vi "IMU and RoboteQ.vi"() -> ()   [LabVIEW 2012]
uses:
  LabVIEW Library v2/AHRS/Controls/Desciptor Set Byte.ctl
  <vilib>/Platform/TimedLoop/XDataNode/timing_clust.ctl
  <vilib>/Platform/TimedLoop/XDataNode/nitl_modes.ctl
  <vilib>/Platform/TimedLoop/XDataNode/wakeup.ctl
  <vilib>/FPGAPlugInAG/cRIO-9113/niLvFpga_Open_cRIO-9113.vi
  <vilib>/FPGAPlugInAG/cRIO-9113/niLvFpga_Reset_cRIO-9113.vi
  <vilib>/FPGAPlugInAG/cRIO-9113/niLvFpga_Run_cRIO-9113.vi
  <vilib>/Utility/error.llb/Error Cluster From Error Code.vi
  <vilib>/RVI Host/nirviSupport.llb/nirviErrorClusterFromErrorCode.vi
  <vilib>/rvi/errors/niLvFpgaAdjustHostInterfaceError.vi
  <vilib>/Instr/_visa.llb/VISA Configure Serial Port (Instr).vi
  LabVIEW Library v2/AHRS/SubVI/3DM-GX3-45 Commands/Start Stream.vi
  LabVIEW Library v2/AHRS/SubVI/3DM-GX3-45 Commands/Stop Stream.vi
  <vilib>/Platform/TimedLoop/XDataNode/XDataNode.xnode
  <vilib>/rvi/interface/nirviOpenFPGA/nirviOpenFPGA.xnode
  FPGA Bitfiles/NI-987xSerialLoo_FPGATarget4_9870InterfaceDMA_U4jeboZBP6A.lvbitx
  Program Files (x86)/National Instruments/LabVIEW 2012/examples/CompactRIO/Module Specific/NI 987x/Serial Loopback/VIs/9870 Interface DMA (FPGA).vi
  <vilib>/rvi/interface/nirviMethod/nirviMethod.xnode
  Labview/Roboteq.lvlib
  <vilib>/Platform/TimedLoop/XDataNode/XDNodeRunTimeDep.lvlib
  Labview/Public/Set Control Effort.vi
  <vilib>/rvi/interface/nirviMethod/StockFPGA_InlinedMethodWaitForSingleIRQ.vi
  <vilib>/FPGAPlugInAG/cRIO-9113/niLvFpga_WaitOnIrq_cRIO-9113.vi
panel:
  out "Byte Count":u32
  out "Read Bytes":string
  out "result":bool
  in  "IMU VISA":refnum<visa-resource-name>="COM5"
  out "Error Out":errorcluster
  in  "Error In":errorcluster
  out "Received Array":u8[](array[numeric]) format="%02x"
  out "Processing Loop Count":i32
  out "Received array Size":i32
  out "YAW":dbl(knob) scale=-180.0..180.0
  out "result string":string
  out "Read Loop Count":i32
  in  "Stop Data Stream":bool
  in  "Start Data Stream":bool
  in  "Self Test":bool
  out "Serial Settings:Number of Bytes at Serial Port":u32
  out "timed out?":bool
  in  "Field Data":u8[](array[numeric]) format="%02x"
  in  "Field Descriptor Byte":u8=117 format="%02x"
  in  "Data Set":T1=enum."NAV"
  in  "ID Query (True)":bool=TRUE
  in  "Motor1 Effort":i32(slide) scale=-10.0..10.0
  in  "Motor2 Effort":i32(slide) scale=-10.0..10.0
  in  "End Loop":bool
  in  "stop?":bool
  out "Telemetry":T2={"Voltage"={0.0, 0.0, 0.0}, "Encoder Speed"={0, 0}, "Temps"={"IC Temp (C)"=0, "Ch1 Temp (C)"=0, "Ch2 Temp (C)"=0}, "Current"={0.0, 0.0, 0.0, 4.6238981750249924e+36}} {"Current" scale=0.0..16.0; "Temps"."IC Temp (C)" scale=0.0..150.0; "Temps"."Ch1 Temp (C)" scale=0.0..150.0; "Temps"."Ch2 Temp (C)" scale=0.0..150.0; "Encoder Speed" scale=-100.0..100.0; "Voltage" scale=8.0..14.0}
  out "Command to Serial":string
  in  "RoboteQ VISA":refnum<visa-resource-name>
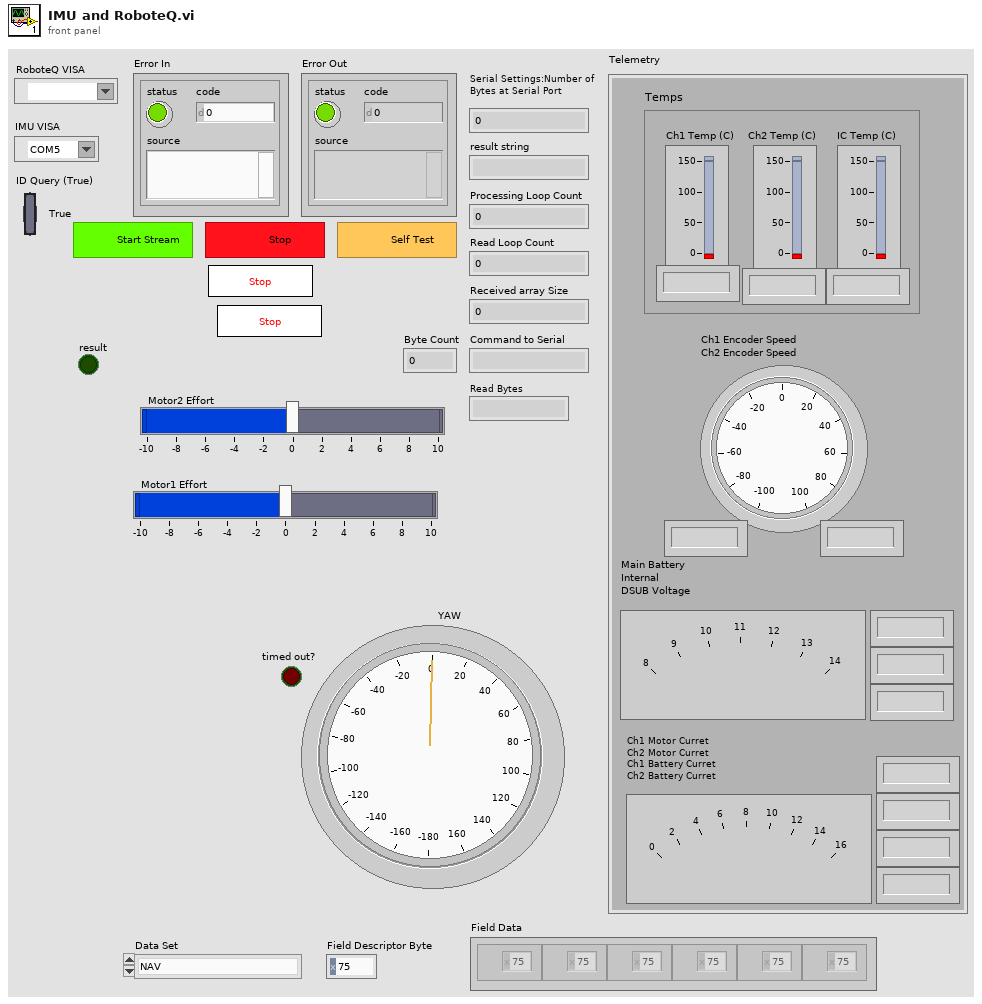
[diagram p1: front panel]
types:
  T1 = typedef "Desciptor Set Byte.ctl" = enum16{"Base Command Set", "3DM Command Set", "Navigation Filter Command Set", "System Command Set", "AHRS", "GPS", "NAV"}
  T2 = cluster{"Voltage":cluster{sgl, sgl, sgl}, "Encoder Speed":cluster{i32, i32}, "Temps":cluster{"IC Temp (C)":i32, "Ch1 Temp (C)":i32, "Ch2 Temp (C)":i32}, "Current":cluster{dbl, dbl, dbl, dbl}}
  T3 = typedef "XDNodeRunTimeDep.lvlib/timing_clust.ctl" = cluster{"Expected End [f-1]":u64, "Actual End [f-1]":u64, "Finished Late? [f-1]":bool, "Expected End [i-1]":u64, "Actual End [i-1]":u64, "Finished Late? [i-1]":bool, "Expected Start [i]":u64, "Actual Start [i]":u64, "Expected Start [f]":u64, "Actual Start [f]":u64, "Source Name":string, "Structure Name":string, "Period":i64, "Deadline":i64, "Offset":i64, "Start":i64, "Priority":i32, "Timeout":i32, "Mode":T4, "Wakeup Reason":T5, "Error":errorcluster, "Source Type":string, "Secondary Source Type":string, "Global End Time":u64, "Global Start Time":u64, "Frame Duration":u64, "Iteration Duration":u64, "Assigned CPU":i32, "I/O Scan Engine Mode":u32}
  T4 = typedef "XDNodeRunTimeDep.lvlib/nitl_modes.ctl" = enum32{"No Change", "Process missed periods, maintain original phase", "Discard missed periods, maintain original phase", "Process missed periods, ignore original phase", "Discard missed periods, ignore original phase"}
  T5 = typedef "XDNodeRunTimeDep.lvlib/wakeup.ctl" = enum32{"Normal", "Aborted", "Asynchronous wakeup", "Timing source error", "Timed loop error", "Timeout"}
  T6 = typedef "901x DMA FPGA Reference.ctl" = refnum<k20>
  T7 = cluster{"main battery voltage (V)":sgl, "internal voltage (V)":sgl, "DSUB voltage (V)":sgl}
  T8 = cluster{" Ch1  Motor current (I)":sgl, " Ch2 Motor current (I)":sgl, " Ch1 Battery current (I)":sgl, " Ch2 Battery current (I)":sgl}
  T9 = cluster{"Ch1 Temp (C)":i32, "Ch2 Temp (C)":i32, "IC Temp (C)":i32}
  T10 = cluster{"Encoder Speed (RPM)":i32, "Encoder Speed (RPM)":i32}
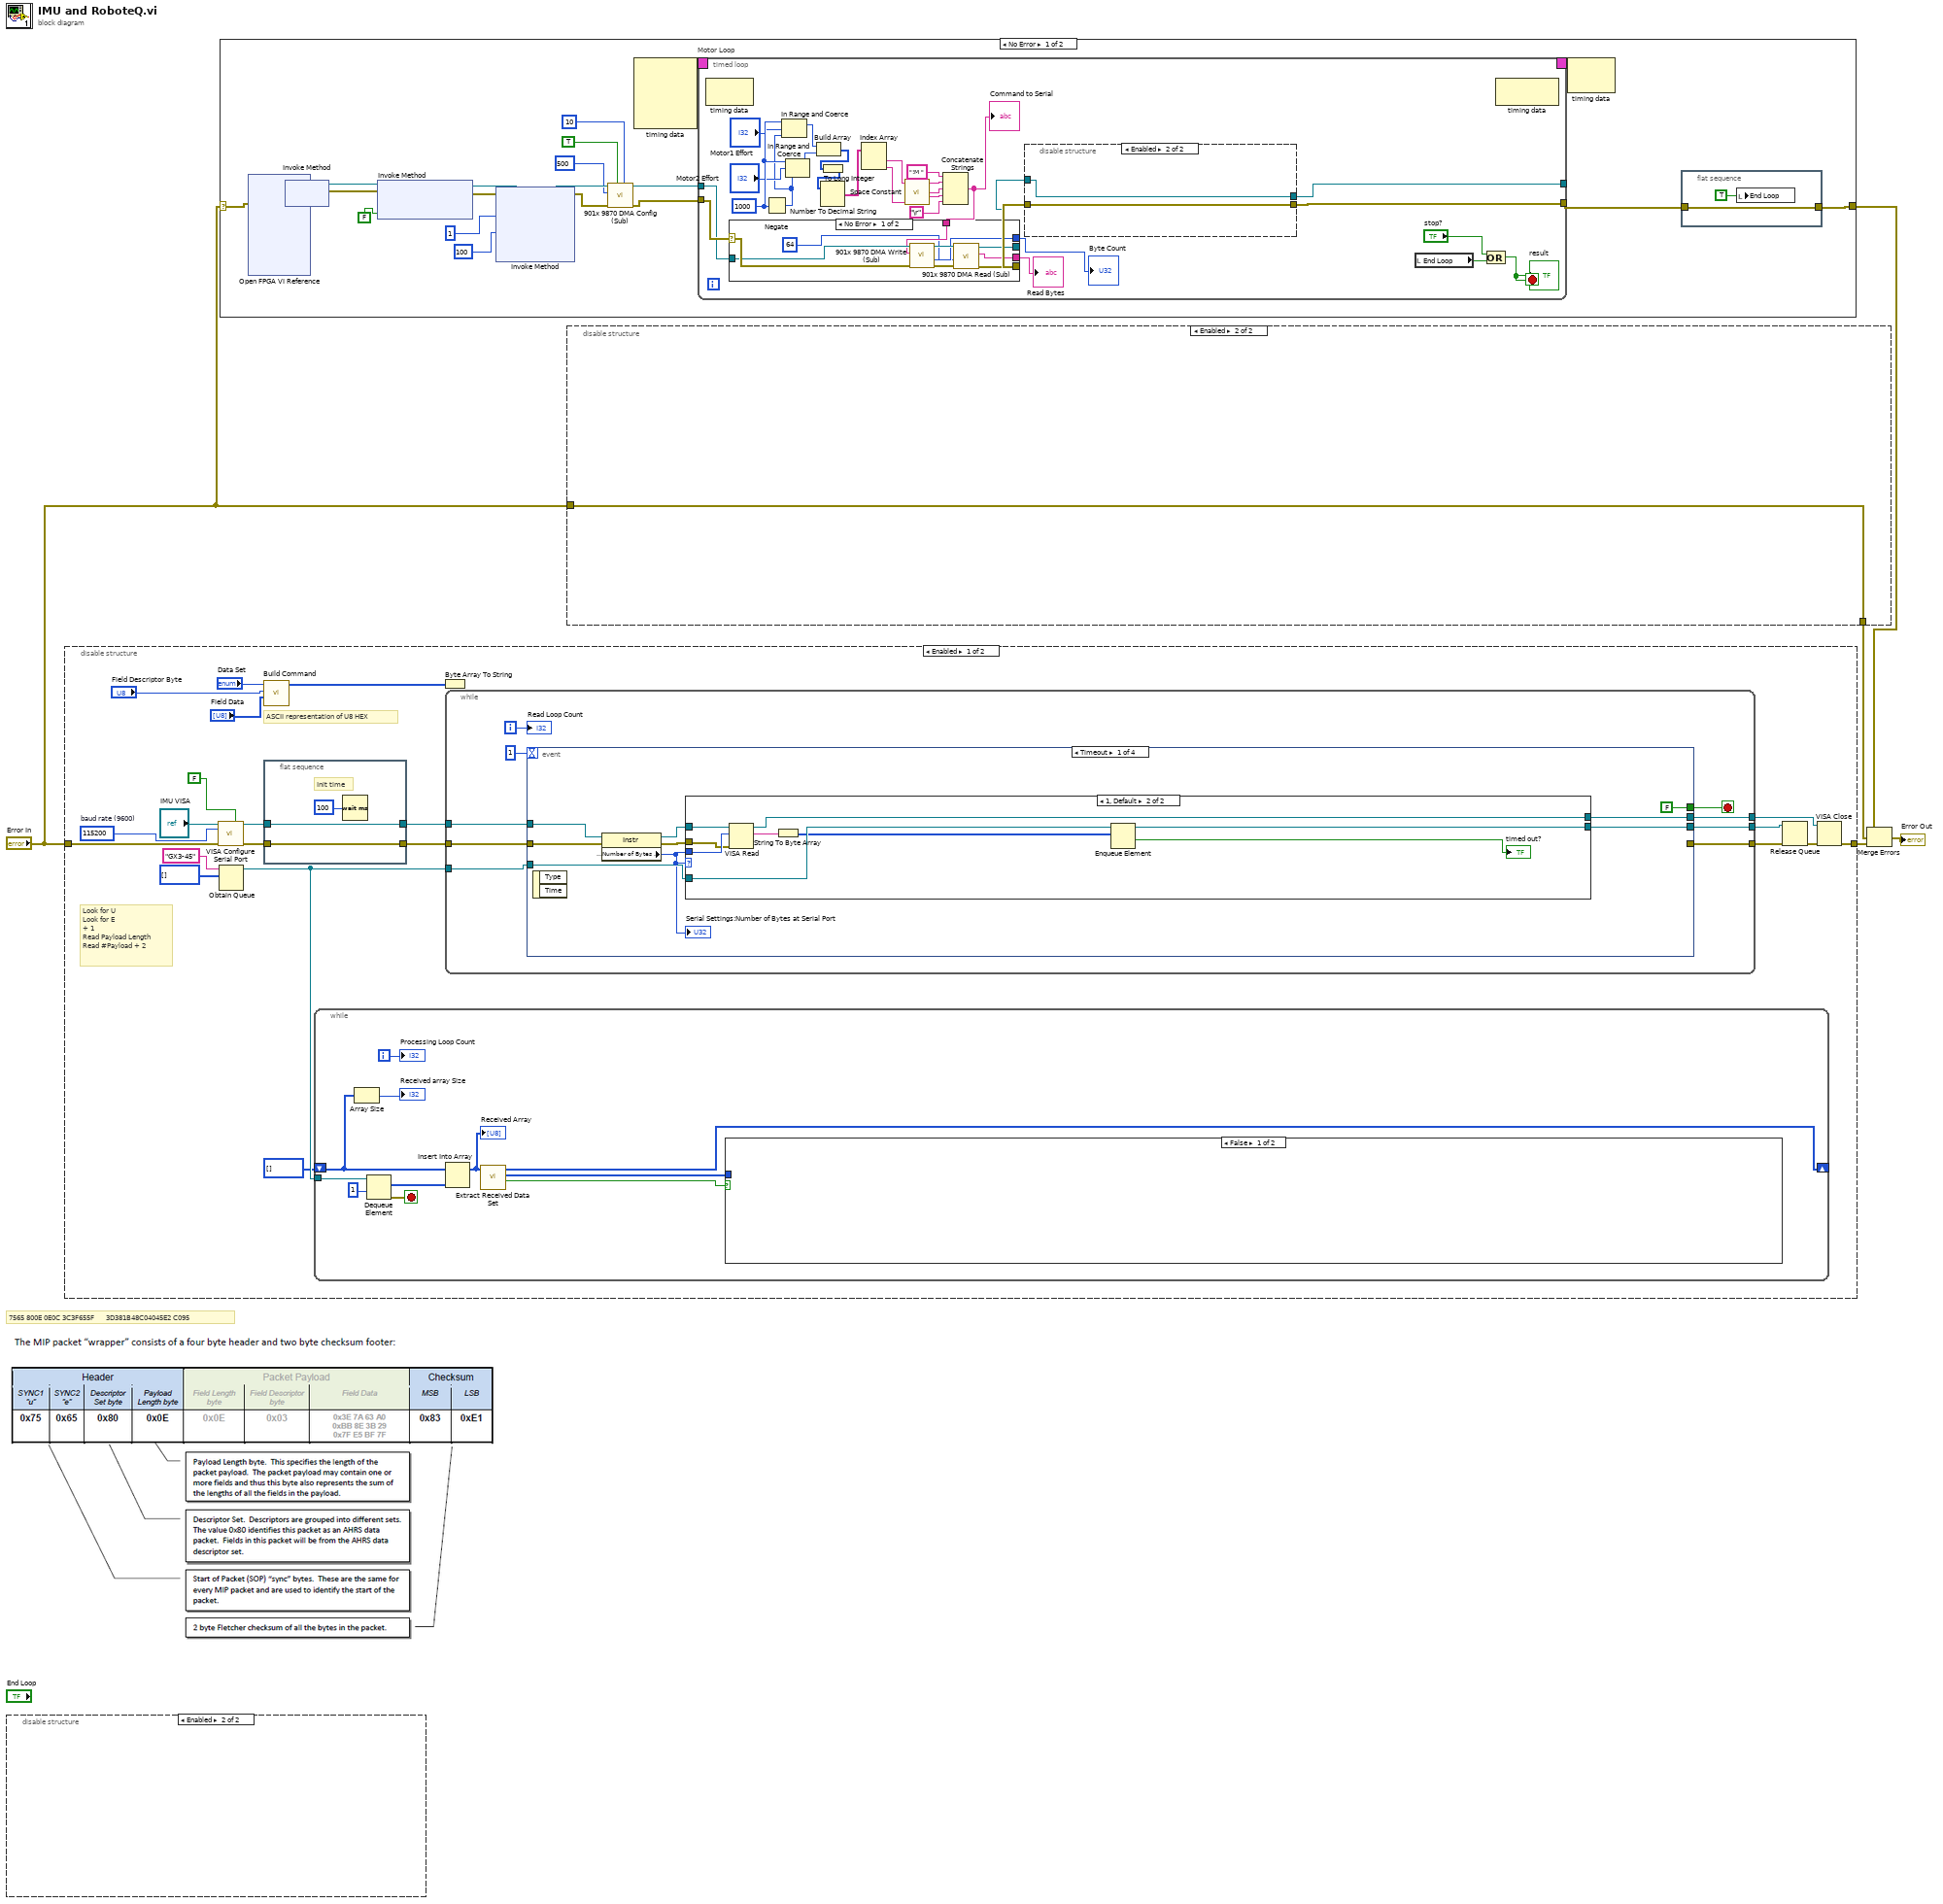
[diagram p0: block diagram]
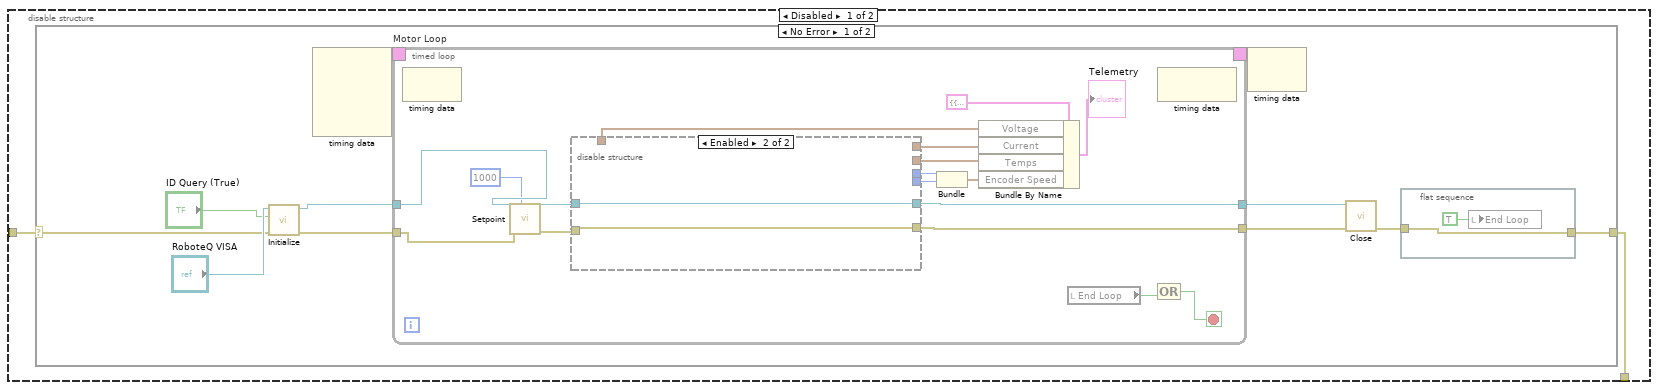
[diagram p2: hidden frame]
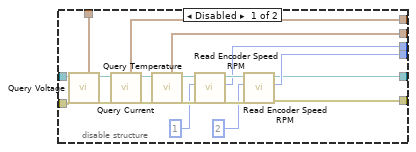
[diagram p3: hidden frame]
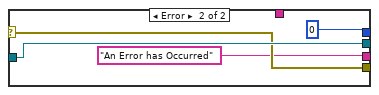
[diagram p5: hidden frame]
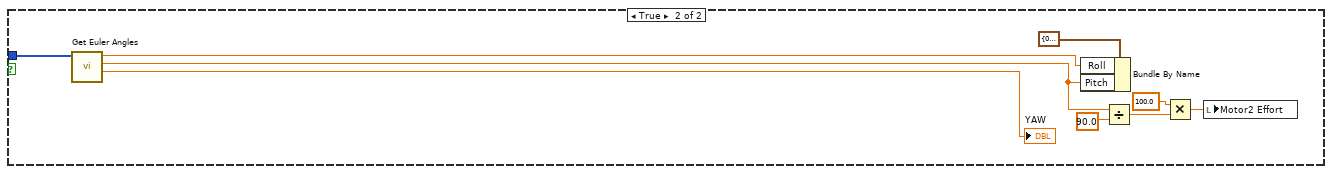
[diagram p8: hidden frame]
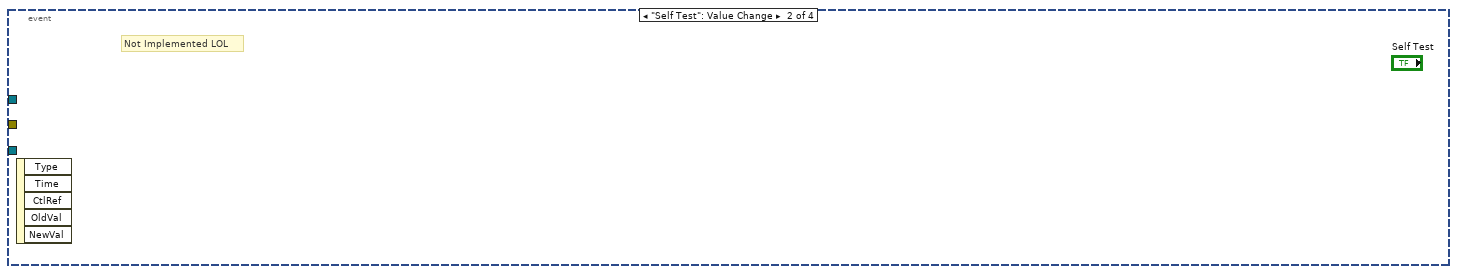
[diagram p10: hidden frame]
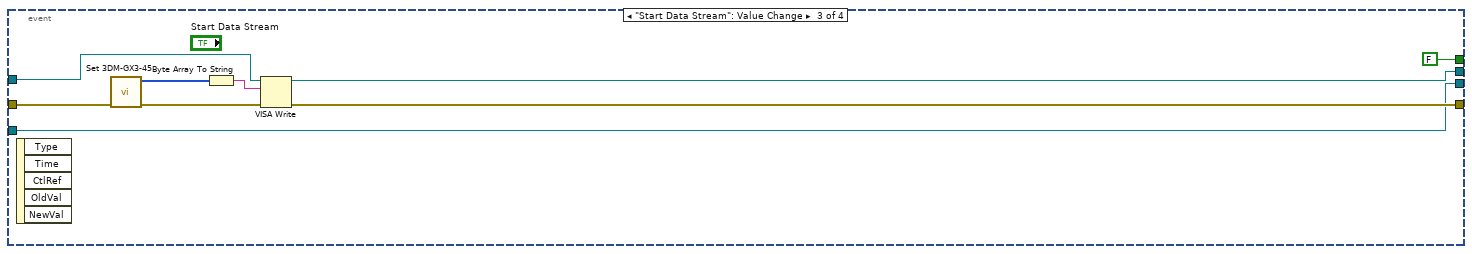
[diagram p11: hidden frame]
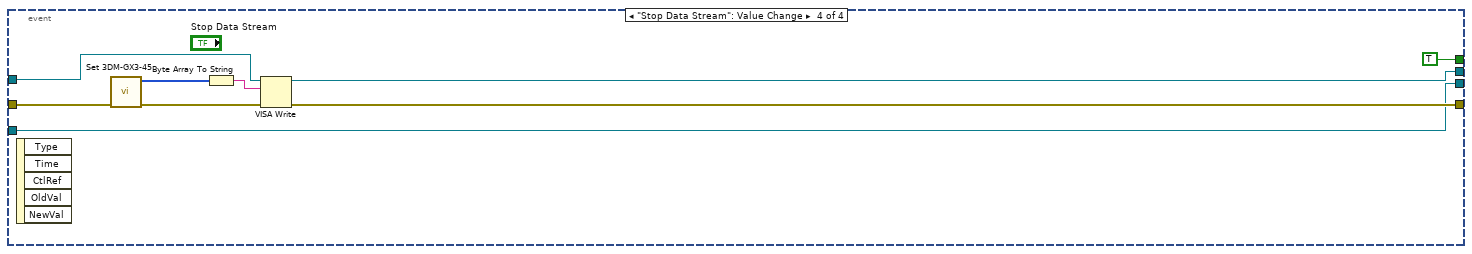
[diagram p12: hidden frame]
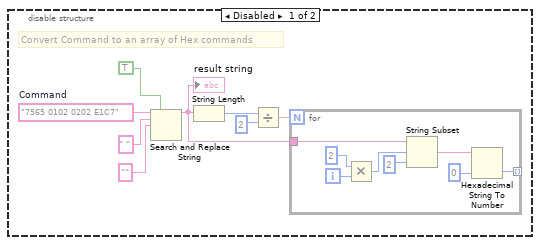
[diagram p14: hidden frame]
diagram:
  # "7565 800E 0E0C 3C3F655F      3D381B48C04045E2 C095"
  n1 = disable-structure shown="Enabled" {
    frame Disabled {
      w13 = "7565 0102 0202 E1C7"  # Command
      # "Convert Command to an array of Hex commands"
      n2 = Search and Replace String(replace all?=TRUE ("replace all? (F)"), input string=w13, search string=" ", replace string="" ("replace string (\"\")")) -> (result string=w9:string)  [unwired: 4 in, 3 out]
      "result string" <- w9
      n3 = String Length(string=w9) -> (length=w8:i32)
      n4 = Divide(x=w8, y=2) -> (x/y=w6:dbl)
      n5 = for {
        N: w6 -> [_]
        tunnel: w9 -> [w21]
        tunnel: [w14] -> _ mode=indexing
        i -> [w19]
        n6 = Multiply(x=2, y=w19) -> (x*y=w17:i32)
        n7 = String Subset(string=w21, offset (0)=w17, length (rest)=2 ("length (rest)")) -> (substring=w16:string)
        n8 = Hexadecimal String To Number(string=w16, default (0uL)=u8 0 ("default (0 U32)")) -> (number=w14:u8)  [unwired: 1 in, 1 out]
      }
    }
    frame Enabled {
    }
  }
  n9 = disable-structure shown="Enabled" {
    disable-tunnel: [w23 w113] -> w3
    disable-tunnel: "Error In" -> [w22 w113]
    frame Enabled {
      w38 = u32 115200  # baud rate (9600)
      # "Look for U\nLook for E\n+ 1\nRead Payload Length\nRead #Payload + 2"
      # "ASCII representation of U8 HEX"
      n10 = call-poly "VISA Configure Serial Port"("VISA resource name"="IMU VISA", "Enable Termination\nChar (T)"=FALSE ("Enable Termination\nChar (T)"), "baud rate (9600)"=w38, "error in (no error)"=w22) -> ("VISA resource name out"=w28:refnum<visa-resource-name>, "error out"=w25:errorcluster)  [unwired: 10 in]
      n11 = Obtain Queue(name (unnamed)="GX3-45", element data type=u8[] [] ("unsigned byte array")) -> (queue out=w31:refnum<queue>)  [unwired: 3 in, 2 out]
      n12 = call "Build Command.vi"("Field Data"="Field Data", "Field Descriptor Byte"="Field Descriptor Byte", "Data Set"="Data Set") -> ("Command"=w34:u8[])  [unwired: 7 in, 1 out]
      n13 = flat-sequence {
        tunnel: w28 -> [w112]
        tunnel: [w112] -> w37
        tunnel: w25 -> [w110]
        tunnel: [w110] -> w24
        frame #0 {
          # "Init time"
          n14 = Wait (ms)(milliseconds to wait=u32 100) -> ()  [unwired: 1 out]
        }
      }
      n15 = while {
        tunnel: w31 -> [w53]
        shift-right: [w47] -> _
        shift-left: u8[] [] ("element") -> [w45]
        i -> [w50]
        stop <- w52 stop-if-true
        n16 = Array Size(array=w45) -> (size(s)=→"Received array Size":i32)
        n17 = Dequeue Element(queue=w53, timeout in ms (-1)=1) -> (element=w51:u8[], error out=w52:errorcluster)  [unwired: 1 in, 2 out]
        n18 = Insert Into Array(array=w45, new element=w51) -> (w49:u8[])  [unwired: 1 in]
        "Received Array" <- w49
        n19 = call "Extract Received Data Set.vi"("Received Array In"=w49) -> ("New Data Set Received"=w44:bool, "Extracted Data Set"=w48:u8[], "Received Array Out"=w47:u8[])  [unwired: 7 in, 1 out]
        n20 = case shown="False" w44 {
          tunnel: w48 -> [_ w62]
          frame False {
          }
          frame True {
            n21 = call "Get Euler Angles.vi"("Received Array"=w62) -> ("Yaw (deg)"=→"YAW":dbl, "Pitch (deg)"=w55:dbl, "Roll (deg)"=w59:dbl)  [unwired: 7 in]
            n22 = Bundle By Name(cluster=cluster{"Roll":dbl, "Pitch":dbl} {"Roll"=0.0, "Pitch"=0.0} ("Attitude Indicator 2"), "Roll"=w59, "Pitch"=w55) -> ()  [unwired: 1 out]
            n23 = Divide(x=w55, y=90.0) -> (x/y=w57:dbl)
            n24 = Multiply(x=100.0, y=w57) -> (x*y=w54:dbl)
            n25 = local write "Motor2 Effort"(w54) -> ()
          }
        }
        "Processing Loop Count" <- w50
      }
      n26 = Byte Array To String(unsigned byte array=w34) -> ()  [unwired: 1 out]
      n27 = while {
        tunnel: w37 -> [w71]
        tunnel: [w70] -> w35
        tunnel: w31 -> [w68]
        tunnel: [w67] -> w30
        tunnel: w24 -> [w65]
        tunnel: [w64] -> w27
        i -> [w69]
        stop <- w63 stop-if-true
        n28 = event shown="[0] Timeout" {
          selector: _ -> [_ _ _ _]
          dyn-events: _ -> [_ _ _ _]
          timeout: 1 -> [_ _ _ _]
          tunnel: w71 -> [w80 _ w100 w109]
          tunnel: [w78 _ w97 w106] -> w70
          tunnel: w68 -> [w76 _ w92 w101]
          tunnel: [w74 _ w92 w101] -> w67
          tunnel: w65 -> [w73 _ w96 w105]
          tunnel: [_ _ w94 w103] -> w64
          tunnel: [FALSE ("Stop Data Stream 2") _ FALSE ("Stop Data Stream 2") TRUE ("Stop Data Stream 2")] -> w63
          event Timeout {
            n29 = event-data() -> ()  [unwired: 1 in, 2 out]
            n30 = property class="Instr"(reference=w80, error in=w73) -> (reference out=w79:refnum<visa-resource-name>, error out=w77:errorcluster, "Serial Settings:Number of Bytes at Serial Port"=w75:u32)
            "Serial Settings:Number of Bytes at Serial Port" <- w75
            n31 = case shown="1, Default" w75 {
              tunnel: w79 -> [w82 w91]
              tunnel: [w82 w90] -> w78
              tunnel: w75 -> [_ w89]
              tunnel: w77 -> [_ w88]
              tunnel: w76 -> [w81 w86]
              tunnel: [w81 w83] -> w74
              frame 0 {
              }
              frame 1, Default {
                n32 = VISA Read(VISA resource name=w91, byte count=w89, error in (no error)=w88) -> (VISA resource name out=w90:refnum<visa-resource-name>, read buffer=w87:string)  [unwired: 2 out]
                n33 = String To Byte Array(string=w87) -> (unsigned byte array=w85:u8[])
                n34 = Enqueue Element(queue=w86, element=w85) -> (queue out=w83:refnum<queue>, timed out?=→"timed out?":bool)  [unwired: 2 in, 1 out]
              }
            }
          }
          event "Self Test": Value Change {
            # "Not Implemented LOL"
            n35 = event-data() -> ()  [unwired: 1 in, 5 out]
          }
          event "Start Data Stream": Value Change {
            n36 = event-data() -> ()  [unwired: 1 in, 5 out]
            n37 = call-poly "Set 3DM-GX3-45.vi"("Error In"=w96) -> ("Error Out"=w95:errorcluster, "Command"=w99:u8[])  [unwired: 9 in]
            n38 = Byte Array To String(unsigned byte array=w99) -> (string=w98:string)
            n39 = VISA Write(VISA resource name=w100, write buffer=w98, error in (no error)=w95) -> (VISA resource name out=w97:refnum<visa-resource-name>, error out=w94:errorcluster)  [unwired: 1 out]
          }
          event "Stop Data Stream": Value Change {
            n40 = event-data() -> ()  [unwired: 1 in, 5 out]
            n41 = call-poly "Set 3DM-GX3-45.vi"("Error In"=w105) -> ("Error Out"=w104:errorcluster, "Command"=w108:u8[])  [unwired: 9 in]
            n42 = Byte Array To String(unsigned byte array=w108) -> (string=w107:string)
            n43 = VISA Write(VISA resource name=w109, write buffer=w107, error in (no error)=w104) -> (VISA resource name out=w106:refnum<visa-resource-name>, error out=w103:errorcluster)  [unwired: 1 out]
          }
        }
        "Read Loop Count" <- w69
      }
      n44 = Release Queue(queue=w30, error in (no error)=w27) -> (error out=w26:errorcluster)  [unwired: 1 in, 2 out]
      n45 = VISA Close(VISA resource name=w35, error in (no error)=w26) -> (error out=w23:errorcluster)
    }
    frame Disabled {
    }
  }
  n46 = case shown="No Error" "Error In" {
    selector: "Error In" -> [w131 w183]
    tunnel: [w115 w183] -> w2
    frame No Error {
      n47 = xnode "Open FPGA VI Reference"("error in"=w131) -> ("FPGA VI Reference Out"=w132:refnum<k20>, "error out"=w130:errorcluster)  [unwired: 1 in]
      n48 = xnode "Invoke Method"("FPGA VI Reference In"=w132, "error in"=w130) -> ("FPGA VI Reference Out"=w127:refnum<k20>, "error out"=w128:errorcluster)
      n49 = xnode "Invoke Method"("FPGA VI Reference In"=w127, "error in"=w128, "Wait Until Done (F)"=FALSE) -> ("FPGA VI Reference Out"=w124:refnum<k20>, "error out"=w125:errorcluster)
      n50 = xnode "Invoke Method"("FPGA VI Reference In"=w124, "error in"=w125, "IRQ Number(s)"=1, "Timeout (ms)"=100) -> ("FPGA VI Reference Out"=w120:refnum<k20>, "error out"=w119:errorcluster)  [unwired: 2 out]
      n51 = call "901x 9870 DMA Config (Sub).vi"("EOS Byte"=10, "Enable EOS"=TRUE, "error in"=w119, "Byte Timeout"=500, "FPGA In"=w120) -> ("error out"=w116:errorcluster, "FPGA Out"=w117:T6)  [unwired: 5 in]
      n52 = node-c288() -> (w134:T3)  [unwired: 4 in]
      n53 = timed-loop "Motor Loop" {
        tunnel: [w157] -> w114
        tunnel: [w158] -> _
        timing: w134 -> [_]
        timing-out: [_] -> w133
        tunnel: w117 -> [w153]
        tunnel: w116 -> [w156]
        stop <- w160 stop-if-true
        w155 = 1000 ("Max Effort")
        n54 = node-c288() -> ()  [unwired: 1 in, 1 out]
        n55 = Negate(x=w155) -> (-x=w149:i32)
        n56 = In Range and Coerce(upper limit=w155, x="Motor1 Effort", lower limit=w149) -> (coerced(x)=w148:i32)  [unwired: 1 out]
        n57 = In Range and Coerce(upper limit=w155, x="Motor2 Effort", lower limit=w149) -> (coerced(x)=w147:i32)  [unwired: 1 out]
        n58 = Build Array(w148, w147) -> (w146:i32[])
        n59 = To Long Integer(number=w146) -> (32bit integer=w145:i32[])
        n60 = Number To Decimal String(number=w145) -> (decimal integer string=w144:string[])  [unwired: 1 in]
        n61 = Index Array(array=w144) -> (element #1=w142:string, element #2=w141:string)  [unwired: 2 in]
        n62 = call <vilib>:"Space Constant.vi"() -> ("String"=w152:string)
        n63 = Concatenate Strings("!M " ("string"), w142, w152, w141, "\r") -> (w140:string)
        "Command to Serial" <- w140
        n64 = case shown="No Error" w156 {
          selector: w156 -> [w170 w173]
          tunnel: w153 -> [w169 w174]
          tunnel: [w166 w174] -> w138
          tunnel: [w165 w173] -> w139
          tunnel: w140 -> [w164 _]
          tunnel: [w163 "An Error has Occurred"] -> w136
          tunnel: [w162 0] -> w135
          frame No Error {
            n65 = call "901x 9870 DMA Write (Sub).vi"("error in"=w170, "Send Data"=w164, "FPGA In"=w169) -> ("error out"=w167:errorcluster, "Byte Count"=w162:u32, "FPGA Out"=w168:T6)  [unwired: 4 in, 2 out]
            n66 = call "901x 9870 DMA Read (Sub).vi"("error in"=w167, "Number of bytes"=64, "FPGA In"=w168) -> ("error out"=w165:errorcluster, "Read Bytes"=w163:string, "FPGA Out"=w166:T6)  [unwired: 3 in, 3 out]
          }
          frame Error {
          }
        }
        "Read Bytes" <- w136
        "Byte Count" <- w135
        n67 = disable-structure shown="Enabled" {
          disable-tunnel: w139 -> [_ w176]
          disable-tunnel: [_ w175] -> w158
          disable-tunnel: [_ w176] -> w157
          disable-tunnel: w138 -> [_ w175]
          frame Disabled {
          }
          frame Enabled {
          }
        }
        n68 = local read "End Loop"() -> (w159:bool)
        n69 = Compound Arithmetic op=OR("stop?", w159) -> (w160:bool)
        "result" <- w160
        n70 = node-c288() -> ()  [unwired: 1 in, 1 out]
      }
      n71 = node-c288(w133) -> ()  [unwired: 1 out]
      n72 = flat-sequence {
        tunnel: [w181] -> w115
        tunnel: w114 -> [w181]
        frame #0 {
          n73 = local write "End Loop"(TRUE ("End Loop")) -> ()
        }
      }
    }
    frame Error {
    }
  }
  n74 = disable-structure shown="Enabled" {
    disable-tunnel: [w185 w246] -> w4
    disable-tunnel: "Error In" -> [w184 w246]
    frame Disabled {
      n75 = case shown="No Error" w184 {
        selector: w184 -> [w188 w245]
        tunnel: [w186 w245] -> w185
        frame No Error {
          n76 = call "Initialize.vi"("error in (no error)"=w188, "ID Query (True)"="ID Query (True)", "VISA resource name"="RoboteQ VISA") -> ("error out"=w193:errorcluster, "VISA resource name out"=w194:refnum<visa-resource-name>)  [unwired: 7 in]
          n77 = node-c288() -> (w190:T3)  [unwired: 4 in]
          n78 = timed-loop "Motor Loop" {
            tunnel: w194 -> [w215]
            tunnel: w193 -> [w214]
            tunnel: [w197] -> w192
            tunnel: [w210] -> w196
            timing: w190 -> [_]
            timing-out: [_] -> w189
            stop <- w216 stop-if-true
            n79 = node-c288() -> ()  [unwired: 1 in, 1 out]
            n80 = call-poly "Setpoint.vi"("Max Effort"=1000, "error in (no error)"=w214, "VISA resource name"=w215) -> ("error out"=w211:errorcluster, "Command"=w207:string, "VISA resource name out"=w212:refnum<visa-resource-name>, "Motor2 Effort"=w199:i32, "Motor1 Effort"=w198:i32)  [unwired: 4 in]
            n81 = disable-structure shown="Enabled" {
              disable-tunnel: w212 -> [w236 w238]
              disable-tunnel: w211 -> [w235 w237]
              disable-tunnel: [w230 _] -> w204
              disable-tunnel: [w229 _] -> w203
              disable-tunnel: [w219 w238] -> w210
              disable-tunnel: [w228 _] -> w205
              disable-tunnel: [w218 w237] -> w197
              disable-tunnel: [w227 _] -> w206
              disable-tunnel: [w222 _] -> w201
              frame Disabled {
                n82 = call "Query Voltage.vi"("error in (no error)"=w235, "VISA resource name"=w236) -> ("error out"=w225:errorcluster, "VISA resource name out"=w226:refnum<visa-resource-name>, "Voltages"=w227:T7)  [unwired: 4 in, 3 out]
                n83 = call "Query Current.vi"("error in (no error)"=w225, "VISA resource name"=w226) -> ("error out"=w223:errorcluster, "VISA resource name out"=w224:refnum<visa-resource-name>, "Motor Currents"=w222:T8)  [unwired: 3 in, 4 out]
                n84 = call "Query Temperature.vi"("error in (no error)"=w223, "VISA resource name"=w224) -> ("error out"=w233:errorcluster, "VISA resource name out"=w234:refnum<visa-resource-name>, "Temps"=w228:T9)  [unwired: 4 in, 3 out]
                n85 = call "Read Encoder Speed RPM.vi"("error in (no error)"=w233, "channel number"=u8 1, "VISA resource name"=w234) -> ("error out"=w231:errorcluster, "Encoder Speed (RPM)"=w230:i32, "VISA resource name out"=w232:refnum<visa-resource-name>)  [unwired: 6 in]
                n86 = call "Read Encoder Speed RPM.vi"("error in (no error)"=w231, "channel number"=u8 2, "VISA resource name"=w232) -> ("error out"=w218:errorcluster, "Encoder Speed (RPM)"=w229:i32, "VISA resource name out"=w219:refnum<visa-resource-name>)  [unwired: 6 in]
              }
              frame Enabled {
              }
            }
            n87 = Bundle("Encoder Speed (RPM)"=w204, "Encoder Speed (RPM)"=w203) -> (w202:T10)  [unwired: 1 in]
            n88 = Bundle By Name(cluster=T2 {"Voltage"={0.0, 0.0, 0.0}, "Encoder Speed"={0, 0}, "Temps"={"IC Temp (C)"=0, "Ch1 Temp (C)"=0, "Ch2 Temp (C)"=0}, "Current"={0.0, 0.0, 0.0, 0.0}} ("Telemetry"), "Voltage"=w206, "Current"=w201, "Temps"=w205, "Encoder Speed"=w202) -> (→"Telemetry":T2)
            n89 = local read "End Loop"() -> (w213:bool)
            n90 = node-c288() -> ()  [unwired: 1 in, 1 out]
            n91 = Compound Arithmetic op=OR(w213) -> (w216:bool, w217:bool)
          }
          n92 = node-c288(w189) -> ()  [unwired: 1 out]
          n93 = call "Close.vi"("error in (no error)"=w192, "VISA resource name"=w196) -> ("error out"=w191:errorcluster)  [unwired: 9 in]
          n94 = flat-sequence {
            tunnel: w191 -> [w243]
            tunnel: [w243] -> w186
            frame #0 {
              n95 = local write "End Loop"(TRUE ("End Loop")) -> ()
            }
          }
        }
        frame Error {
        }
      }
    }
    frame Enabled {
    }
  }
  n96 = Merge Errors(w2, w4, w3) -> (→"Error Out":errorcluster)
